vi "CreateConnection.vi"(2 "Truck ID":u8, 3 "Port number\nactuators":u16) -> (1 "COM data":T1)   [LabVIEW 2013]
panel:
  out "error out":errorcluster
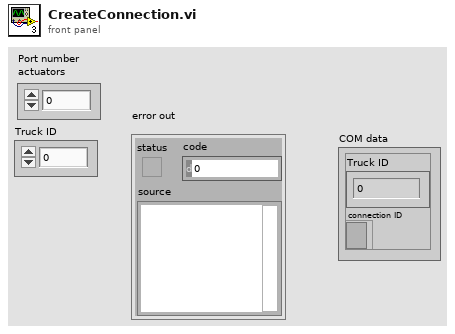
[diagram p1: front panel]
types:
  T1 = cluster{"Truck ID":u8, "connection ID":refnum<k5>}
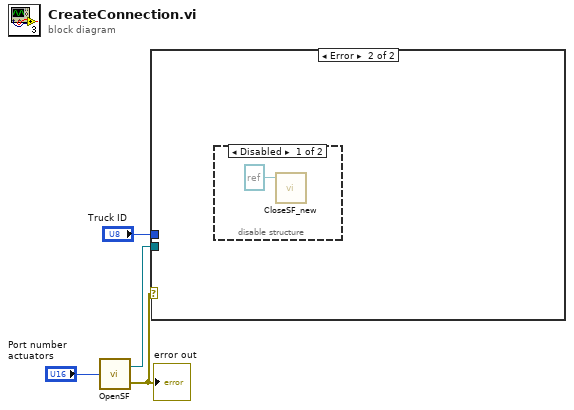
[diagram p0: block diagram]
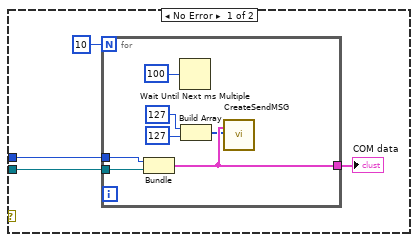
[diagram p2: hidden frame]
diagram:
  n1 = call "OpenSF.vi"("Port number"="Port number\nactuators") -> ("connection ID"=w3:refnum<k5>, "Error out"=w4:errorcluster)
  "error out" <- w4
  n2 = case shown="Error" w4 {
    tunnel: w3 -> [w8 _]
    tunnel: "Truck ID" -> [w6 _]
    frame No Error {
      n3 = for {
        N: 10 -> [_]
        tunnel: w8 -> [w13]
        tunnel: w6 -> [w14]
        tunnel: [w12] -> w5
        n4 = Bundle("Truck ID"=w14, "connection ID"=w13) -> (w12:T1)  [unwired: 1 in]
        n5 = Wait Until Next ms Multiple(millisecond multiple=u32 100) -> ()  [unwired: 1 out]
        n6 = Build Array(u8 127 ("Speed"), u8 127 ("Steering")) -> (w9:u8[])
        n7 = call "CreateSendMSG.vi"("COM Data"=w12, "Controls"=w9) -> ()  [unwired: 18 in]
      }
      "COM data" <- w5
    }
    frame Error {
      n8 = disable-structure shown="Disabled" {
        frame Disabled {
          n9 = call "CloseSF_new.vi"("connection ID"=refnum<k5> refnum) -> ()  [unwired: 2 in]
        }
        frame Enabled {
        }
      }
    }
  }
